vi "Write ids.vi"(8 "error in (no error)":errorcluster, 10 "ids":string, 11 "JSON-RPC in":refnum<class "JSON-RPC.lvclass">) -> (0 "error out":errorcluster, 3 "JSON-RPC out":refnum<class "JSON-RPC.lvclass">)   [LabVIEW 2019, in "JSON-RPC.lvclass"]
uses:
  JSON-RPC.lvclass
  JSON-RPC.lvclass/JSON-RPC.ctl
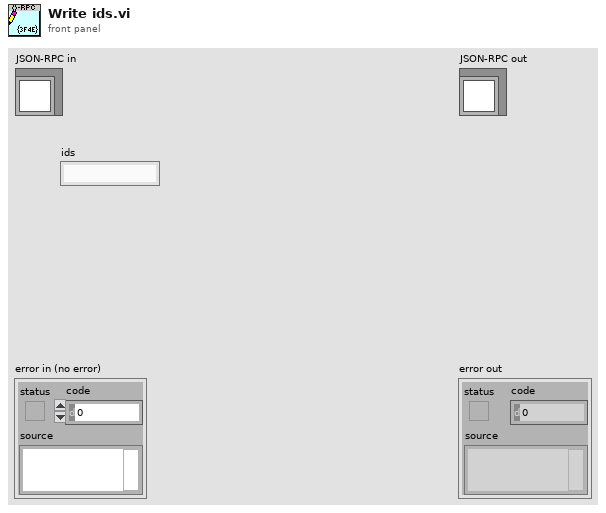
[diagram p1: front panel]
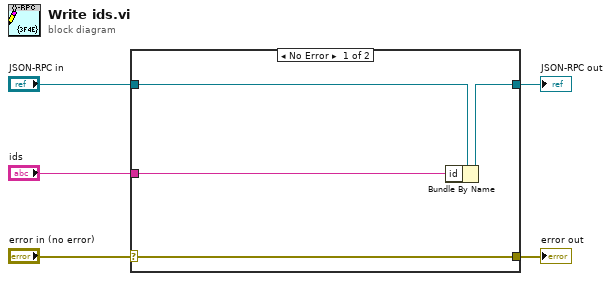
[diagram p0: block diagram]
diagram:
  n1 = case shown="No Error" "error in (no error)" {
    selector: "error in (no error)" -> [w9 w10]
    tunnel: [w9 w10] -> w4
    tunnel: [w6 w11] -> w2
    tunnel: "JSON-RPC in" -> [w8 w11]
    tunnel: "ids" -> [w7 _]
    frame No Error {
      n2 = Bundle By Name(cluster=w8, "id"=w7) -> (w6:refnum<class "JSON-RPC.lvclass">)
    }
    frame Error {
    }
  }
  "error out" <- w4
  "JSON-RPC out" <- w2
